vi "Add Object Parameter - Null.vi"(8 "error in (no error)":errorcluster, 9 "Name":string, 11 "JSON Tree in (JSON Object)":variant) -> (0 "error out":errorcluster, 3 "JSON Tree out (JSON Object)":variant)   [LabVIEW 2010, in "i3-json.lvlib"]
doc: "Use this template to build a VI to use as a subVI."
uses:
  i3-json.lvlib
  JSON Types/JSON Type.ctl
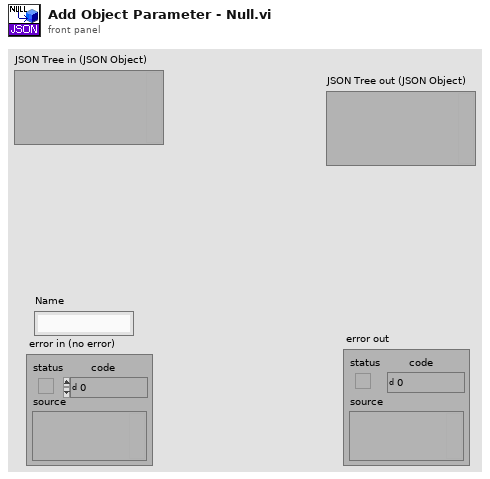
[diagram p1: front panel]
types:
  T1 = typedef "i3-json.lvlib/JSON Type.ctl" = enum8{"JSON Compatible", "JSON Array", "JSON Object", "JSON Null", "Double", "String", "Boolean", "Unknown"}
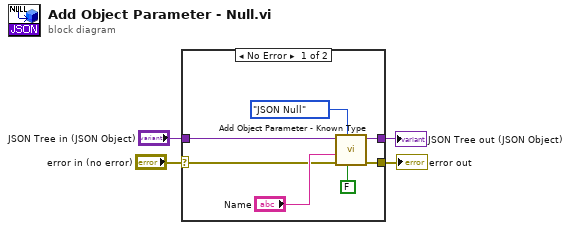
[diagram p0: block diagram]
diagram:
  n1 = case shown="No Error" "error in (no error)" {
    selector: "error in (no error)" -> [w5 w13]
    tunnel: [w11 w13] -> w3
    tunnel: [w10 w12] -> w2
    tunnel: "JSON Tree in (JSON Object)" -> [w9 w12]
    frame No Error {
      n2 = call "Add Object Parameter - Known Type.vi"("Add Parameter as JSON Tree?"=FALSE, "JSON Type"=JSON_Type."JSON Null", "error in (no error)"=w5, "Name"="Name", "JSON Tree in (JSON Object)"=w9) -> ("error out"=w11:errorcluster, "JSON Tree out (JSON Object)"=w10:variant)  [unwired: 5 in]
    }
    frame Error {
    }
  }
  "error out" <- w3
  "JSON Tree out (JSON Object)" <- w2
